vi "axex_create_sheet.vi"(5 "activate sheet (False)":bool, 7 "select new sheet (False)":bool, 8 "error in":errorcluster, 9 "position index (-1: last)":i32=-1, 10 "new sheet name":string, 11 "AX Excel instance in":T1) -> (0 "error out":errorcluster, 3 "AX Excel instance out":T1)   [LabVIEW 2020, in "AX Excel.lvlib"]
doc: "Call this to create new sheet in current excel file. New sheet can be optionally selected and/or activated.\nOption 'position index' sets the position of new sheet in sheets list. Use -1 to place it to the end of list (default), 0 to place it to begining."
uses:
  AX Excel.lvlib
  axex_instance.ctl
  <vilib>/Utility/error.llb/Error Cluster From Error Code.vi
  <vilib>/ErrorRing/Error Ring.xnode
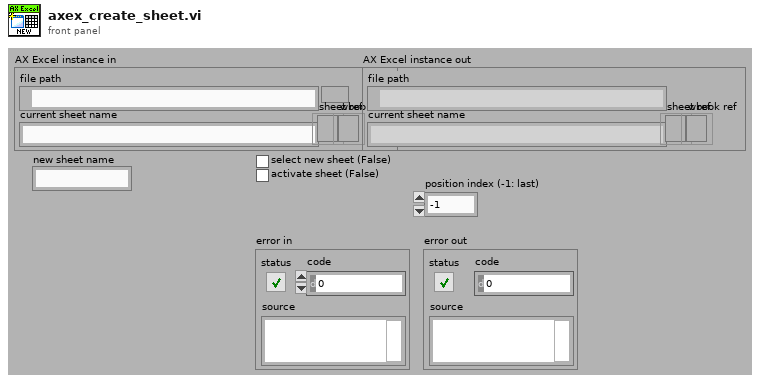
[diagram p1: front panel]
types:
  T1 = typedef "AX Excel.lvlib/axex_instance.ctl" = cluster{"file path":path, "current sheet name":string, "sheet ref":refnum<k7>, "wbook ref":refnum<k7>}
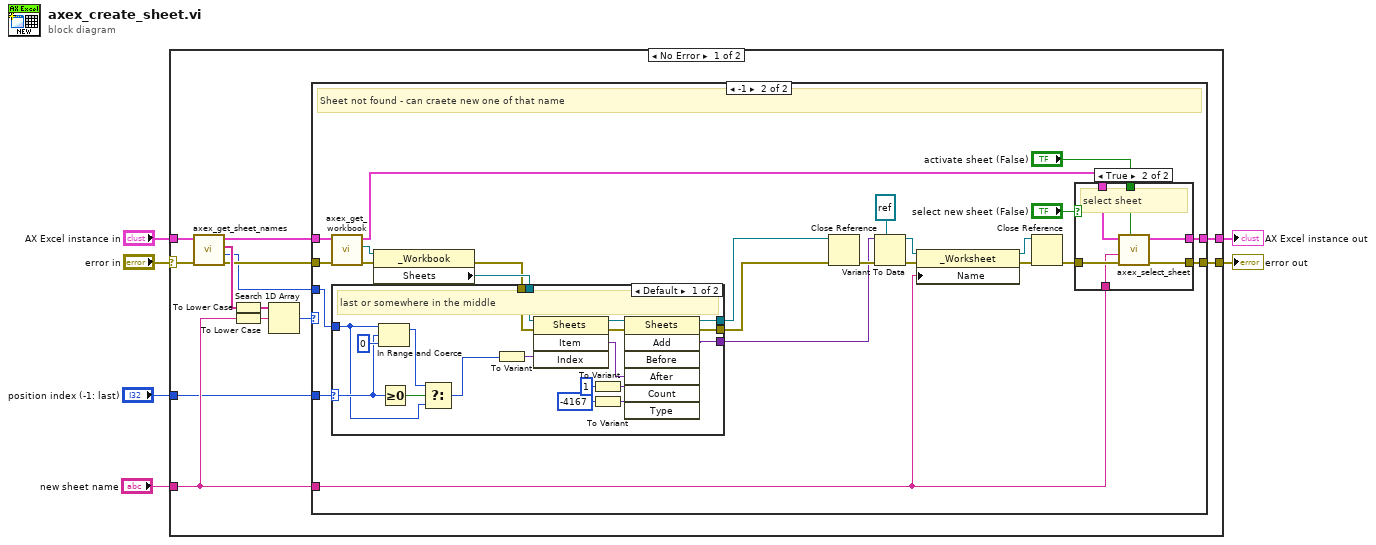
[diagram p0: block diagram]
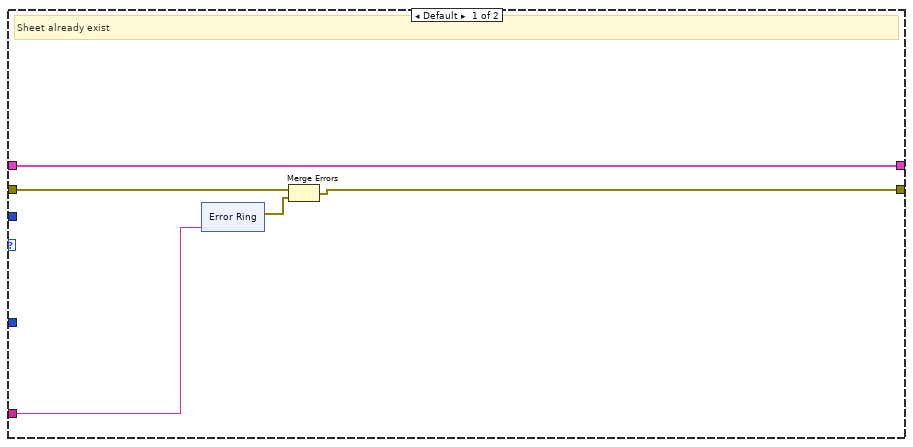
[diagram p2: hidden frame]
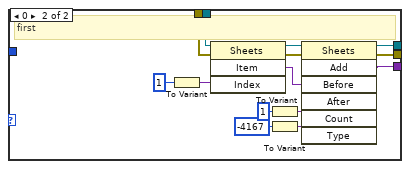
[diagram p3: hidden frame]
diagram:
  n1 = case shown="No Error" "error in" {
    selector: "error in" -> [w7 w98]
    tunnel: "AX Excel instance in" -> [w19 w97]
    tunnel: "new sheet name" -> [w12 _]
    tunnel: [w11 w97] -> w4
    tunnel: [w10 w98] -> w3
    tunnel: "position index (-1: last)" -> [w8 _]
    frame No Error {
      n2 = call "axex_get_sheet_names.vi"("error in"=w7, "AX Excel instance in"=w19) -> ("error out"=w14:errorcluster, "sheets count"=w9:i32, "sheet names"=w18:string[], "AX Excel instance out"=w13:T1)  [unwired: 5 in, 1 out]
      n3 = To Lower Case(string=w18) -> (all lower case string=w17:string[])
      n4 = To Lower Case(string=w12) -> (all lower case string=w16:string)
      n5 = Search 1D Array(1D array=w17, element=w16) -> (index of element=w15:i32)  [unwired: 1 in]
      n6 = case shown="-1" w15 {
        tunnel: w14 -> [w22 w55]
        tunnel: w13 -> [w24 w54]
        tunnel: w12 -> [w23 w43]
        tunnel: [w24 w42] -> w11
        tunnel: [w20 w41] -> w10
        tunnel: w9 -> [_ w37]
        tunnel: w8 -> [_ w38]
        frame Default {
          # "Sheet already exist"
          n7 = xnode "Error Ring"("parameter 0"=w23) -> ("error out"=w21:errorcluster)
          n8 = Merge Errors(w22, w21) -> (w20:errorcluster)
        }
        frame -1 {
          # "Sheet not found - can craete new one of that name"
          n9 = call "axex_get_workbook.vi"("error in"=w55, "AX Excel instance in"=w54) -> ("error out"=w53:errorcluster, "excel workbook"=w52:refnum<k7>, "AX Excel instance out"=w44:T1)  [unwired: 7 in]
          n10 = property class="_Workbook"(reference=w52, error in=w53) -> (error out=w32:errorcluster, "Sheets"=w36:refnum<k7>)  [unwired: 1 out]
          n11 = case shown="Default" w38 {
            selector: w38 -> [w61 _]
            tunnel: w37 -> [w56 _]
            tunnel: w32 -> [w73 w75]
            tunnel: [w63 w84] -> w34
            tunnel: w36 -> [w72 w76]
            tunnel: [w62 w83] -> w35
            tunnel: [w57 w82] -> w33
            frame Default {
              # "last or somewhere in the middle"
              n12 = In Range and Coerce(upper limit=w56, x=w61, lower limit=0) -> (coerced(x)=w59:i32)  [unwired: 1 out]
              n13 = Greater Or Equal To 0?(x=w61) -> (x >= 0?=w60:bool)
              n14 = Select(t=w59, s=w60, f=w56) -> (s? t:f=w58:i32)
              n15 = To Variant(anything=w58) -> (Variant=w71:variant)
              n16 = invoke class="Sheets" method="Item"(reference=w72, error in=w73, "Index"=w71) -> (reference out=w65:refnum<k7>, error out=w66:errorcluster, "Item"=w64:variant)  [unwired: 1 in, 1 out]
              n17 = To Variant(anything=1) -> (Variant=w67:variant)
              n18 = To Variant(anything=-4167) -> (Variant=w70:variant)
              n19 = invoke class="Sheets" method="Add"(reference=w65, error in=w66, "After"=w64, "Count"=w67, "Type"=w70) -> (reference out=w62:refnum<k7>, error out=w63:errorcluster, "Add"=w57:variant)  [unwired: 2 in, 4 out]
            }
            frame 0 {
              # "first"
              n20 = To Variant(anything=1) -> (Variant=w78:variant)
              n21 = invoke class="Sheets" method="Item"(reference=w76, error in=w75, "Index"=w78) -> (reference out=w80:refnum<k7>, error out=w81:errorcluster, "Item"=w79:variant)  [unwired: 1 in, 1 out]
              n22 = To Variant(anything=1) -> (Variant=w85:variant)
              n23 = To Variant(anything=-4167) -> (Variant=w88:variant)
              n24 = invoke class="Sheets" method="Add"(reference=w80, error in=w81, "Before"=w79, "Count"=w85, "Type"=w88) -> (reference out=w83:refnum<k7>, error out=w84:errorcluster, "Add"=w82:variant)  [unwired: 2 in, 4 out]
            }
          }
          n25 = Close Reference(reference=w35, error in (no error)=w34) -> (error out=w50:errorcluster)
          n26 = Variant To Data(error in=w50, type=refnum<k7> refnum ("reference out"), Variant=w33) -> (data=w48:refnum<k7>, error out=w49:errorcluster)
          n27 = property class="_Worksheet"(reference=w48, error in=w49, "Name"=w43) -> (reference out=w46:refnum<k7>, error out=w47:errorcluster)
          n28 = Close Reference(reference=w46, error in (no error)=w47) -> (error out=w45:errorcluster)
          n29 = case shown="True" "select new sheet (False)" {
            tunnel: w45 -> [w90 w96]
            tunnel: w44 -> [w89 w95]
            tunnel: [w90 w94] -> w41
            tunnel: w43 -> [_ w93]
            tunnel: [w89 w92] -> w42
            tunnel: "activate sheet (False)" -> [_ w91]
            frame False {
              # "don't select sheet"
            }
            frame True {
              # "select sheet"
              n30 = call "axex_select_sheet.vi"("activate sheet (False)"=w91, "error in"=w96, "sheet name (none)"=w93, "AX Excel instance in"=w95) -> ("error out"=w94:errorcluster, "AX Excel instance out"=w92:T1)  [unwired: 4 in, 2 out]
            }
          }
        }
      }
    }
    frame Error {
    }
  }
  "error out" <- w3
  "AX Excel instance out" <- w4
